vi "the effect of capacity fading(subVI).vi"(0 "temperature(ªC) battery not used":dbl, 1 "Time cell\nnot used(months)":dbl, 2 "capacity cell":dbl, 3 "N cycles":dbl, 4 "Cycling\ntemperature\nto K factors":u16) -> (5 "capacity \nusable":dbl)   [LabVIEW 2017]
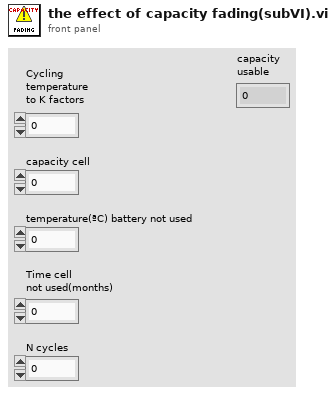
[diagram p1: front panel]
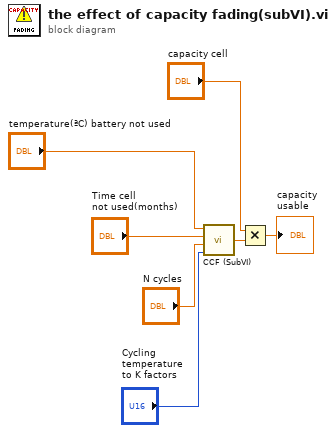
[diagram p0: block diagram]
diagram:
  n1 = call "CCF (SubVI).vi"("Cycling\ntemperature"="Cycling\ntemperature\nto K factors", "N cycles"="N cycles", "Time cell\nnot used(months)"="Time cell\nnot used(months)", "temperature(ªC)"="temperature(ªC) battery not used") -> ("capacity correction factor"=w5:dbl)
  n2 = Multiply(x="capacity cell", y=w5) -> (x*y=→"capacity \nusable":dbl)
